vi "Reverse Waveforms.vi"(1 "signal in":waveform(dbl)[](array[waveform])) -> (0 "Array":waveform(dbl)[](array[waveform]))   [LabVIEW 2019, in "DSP.lvclass"]
uses:
  DSP.lvclass
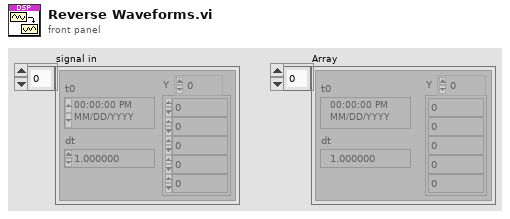
[diagram p1: front panel]
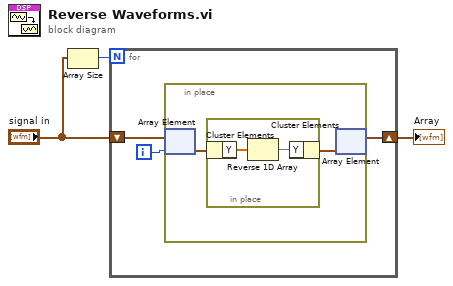
[diagram p0: block diagram]
diagram:
  n1 = Array Size(array="signal in") -> (size(s)=w2:i32)
  n2 = for {
    N: w2 -> [_]
    shift-right: [w4] -> w3
    shift-left: "signal in" -> [w6]
    i -> [w5]
    n3 = in-place {
      n4 = in-place-array #1(w6, w5) -> (w8:waveform(dbl))
      n5 = in-place {
        n6 = in-place-cluster #2(w8) -> ("Y"=w10:dbl[])
        n7 = Reverse 1D Array(array=w10) -> (reversed array=w9:dbl[])
        n8 = in-place-cluster #2("Y"=w9) -> (w7:waveform(dbl))
      }
      n9 = in-place-array #1(w7) -> (w4:waveform(dbl)[])  [unwired: 1 out]
    }
  }
  "Array" <- w3
